vi "Client.vi"() -> ()   [LabVIEW 2016]
uses:
  C:/Users/Administrator/Desktop/HslCommunicationDemo-v5.7.0/HslCommunication.dll
  HslCommunication.dll
panel:
  in  "停止按钮":bool
  out "字符串":string
  out "IsSuccess":bool
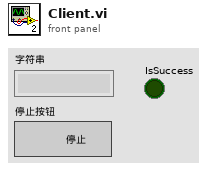
[diagram p1: front panel]
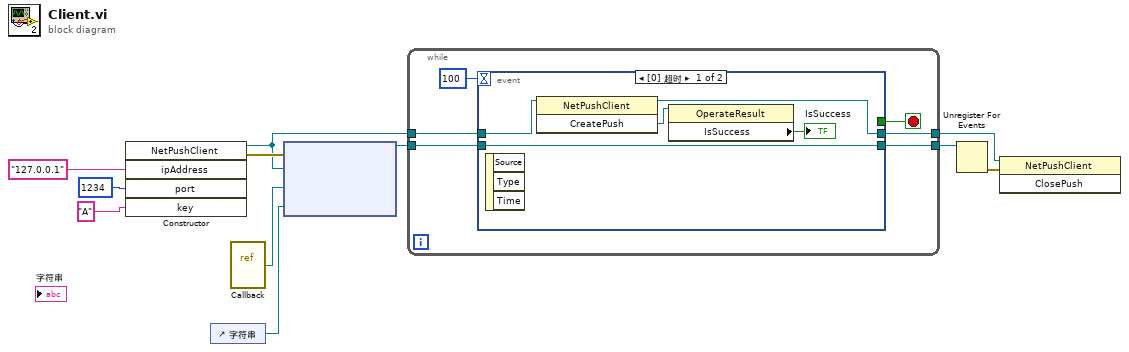
[diagram p0: block diagram]
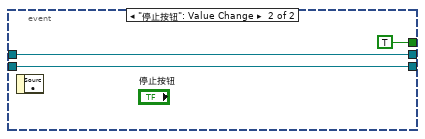
[diagram p2: hidden frame]
diagram:
  n1 = constructor class="NetPushClient"("ipAddress"="127.0.0.1", "port"=1234, "key"="A") -> (reference out=w6:refnum<k24>, error out=w7:errorcluster)  [unwired: 3 in, 4 out]
  n2 = control-ref of="字符串"() -> (w3:refnum<vi>)
  n3 = vi-ref "Callback.vi"() -> ("vi reference"=w2:refnum<vi>)
  n4 = node(w7, w6, w2, w3) -> (w8:refnum<k27>)  [unwired: 1 in, 1 out]
  n5 = while {
    tunnel: w8 -> [w17]
    tunnel: w6 -> [w16]
    tunnel: [w15] -> w5
    tunnel: [w14] -> w4
    stop <- w13 stop-if-true
    n6 = event shown="[0] 超时" {
      selector: _ -> [_ _]
      dyn-events: _ -> [_ _]
      timeout: 100 -> [_ _]
      tunnel: w17 -> [w22 w25]
      tunnel: [w22 w25] -> w14
      tunnel: w16 -> [w19 w24]
      tunnel: [w18 w24] -> w15
      tunnel: [_ TRUE] -> w13
      event Timeout {
        n7 = event-data() -> ()  [unwired: 1 in, 3 out]
        n8 = invoke class="NetPushClient" method="CreatePush"(reference=w19) -> (reference out=w18:refnum<k24>, "CreatePush"=w21:refnum<k24>)  [unwired: 2 in, 1 out]
        n9 = property class="OperateResult"(reference=w21) -> ("IsSuccess"=→"IsSuccess":bool)  [unwired: 1 in, 2 out]
      }
      event "停止按钮": Value Change {
        n10 = event-data() -> ()  [unwired: 1 in, 1 out]
      }
    }
  }
  n11 = Unregister For Events(event registration refnum=w4) -> (error out=w1:errorcluster)  [unwired: 1 in]
  n12 = invoke class="NetPushClient" method="ClosePush"(reference=w5, error in=w1) -> ()  [unwired: 1 in, 3 out]
